vi "NI VeriStand - Set Channel Value.vi"   [LabVIEW 2020, in "NI_VS Workspace ExecutionAPI.lvlib"]
doc: "Sets values of channels on the target. You must manually select the polymorphic instance to use."
uses:
  <vilib>/NI VeriStand/Execution/Workspace/NI_VS Workspace ExecutionAPI.lvlib
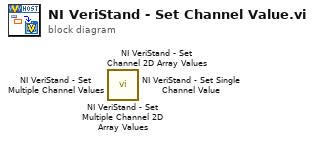
[diagram p0: block diagram]
diagram:
  n1 = call <vilib>:"NI VeriStand - Set Multiple Channel 2D Array Values.vi"() -> ()  [unwired: 10 in, 2 out]
  n2 = call <vilib>:"NI VeriStand - Set Channel 2D Array Values.vi"() -> ()  [unwired: 10 in, 2 out]
  n3 = call <vilib>:"NI VeriStand - Set Multiple Channel Values.vi"() -> ()  [unwired: 10 in, 2 out]
  n4 = call <vilib>:"NI VeriStand - Set Single Channel Value.vi"() -> ()  [unwired: 10 in, 2 out]
